vi "BuildEdgePulse.vi"(4 "输入":bool) -> (0 "下降沿":bool, 1 "输出":bool, 2 "上升沿":bool)   [LabVIEW 2018]
panel:
  out "中间P":bool
  out "中间F":bool
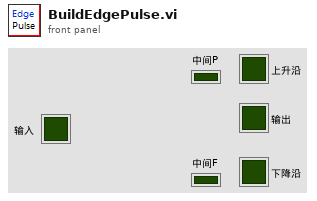
[diagram p1: front panel]
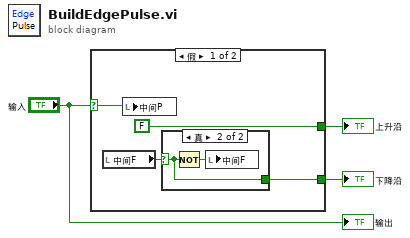
[diagram p0: block diagram]
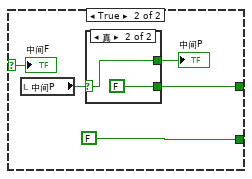
[diagram p3: hidden frame]
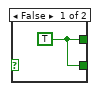
[diagram p4: hidden frame]
diagram:
  n1 = case shown="假" "输入" {
    selector: "输入" -> [w4 w15]
    tunnel: [w6 FALSE] -> w3
    tunnel: [FALSE w12] -> w2
    frame False {
      n2 = local read "中间F"() -> (w7:bool)
      n3 = local write "中间P"(w4) -> ()
      n4 = case shown="真" w7 {
        selector: w7 -> [w8 w9]
        tunnel: [w8 w9] -> w6
        frame False {
        }
        frame True {
          n5 = Not(x=w9) -> (.not. x?=w10:bool)
          n6 = local write "中间F"(w10) -> ()
        }
      }
    }
    frame True {
      n7 = local read "中间P"() -> (w13:bool)
      n8 = case shown="真" w13 {
        selector: w13 -> [_ w17]
        tunnel: [w16 FALSE] -> w12
        tunnel: [w16 w17] -> w11
        frame False {
          w16 = TRUE
        }
        frame True {
        }
      }
      "中间P" <- w11
      "中间F" <- w15
    }
  }
  "下降沿" <- w3
  "上升沿" <- w2
  "输出" <- "输入"
